vi "NDHX.vi"(1 "NDHX Tube Length (m)":dbl, 2 "Pipe Diameter (m)":dbl, 3 "Air Average Viscosity (Pa-s)":dbl, 4 "Thermal Conductivity of FLiNaK (W/m-K)":dbl, 5 "Air Mass Flow (kg/s)":dbl, 6 "Sec Hot Temp (K)":dbl, 9 "Stack Inner Diameter (m)":dbl, 10 "Cp of FLiNaK (J/kgK)":dbl, 11 "Sec Cold Temp (K)":dbl, 12 "NDHX Tube Diameter (m)":dbl, 13 "NDHX Number of Tubes":dbl, 14 "Air Cold Temperature (K)":dbl, 15 "Thermal Conductivity of Hastealloy N (W/m-K)":dbl, 16 "Air Hot Temperature (K)":dbl, 18 "Cp of Air (J/kgK)":dbl, 19 "Sec Mass Flow (kg/s)":dbl) -> (20 "NDHX Heating Transfer (W)":dbl, 21 "Wall Temperature (K)":dbl, 22 "LMTD (K)":dbl)   [LabVIEW 2019]
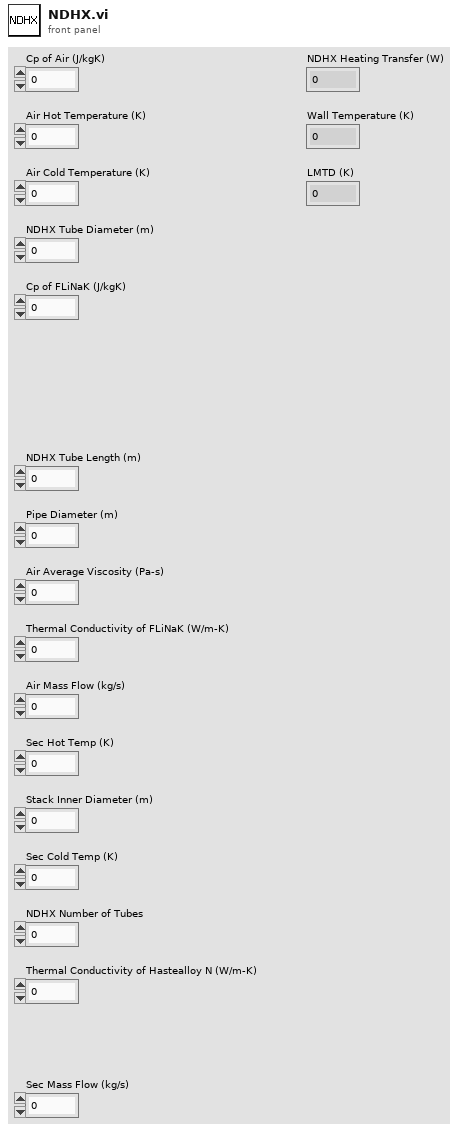
[diagram p1: front panel]
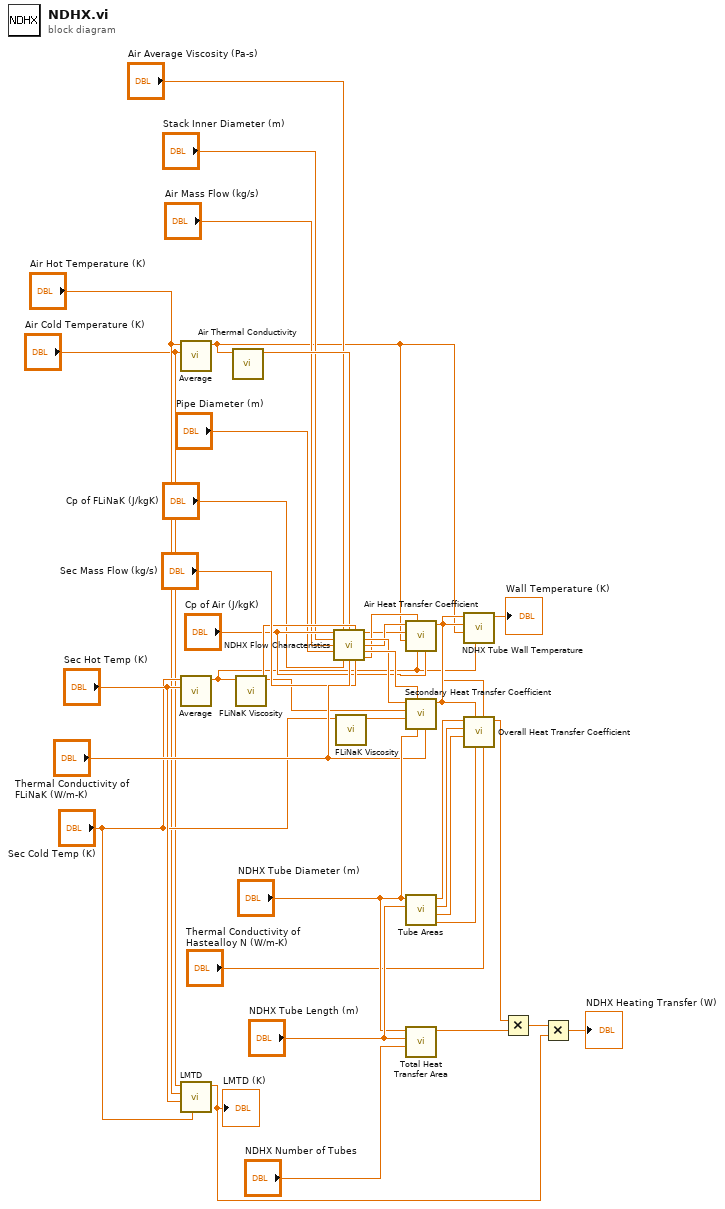
[diagram p0: block diagram]
diagram:
  n1 = call "Average.vi"("Number 2"="Air Cold Temperature (K)", "Number 1"="Air Hot Temperature (K)") -> ("Average"=w1:dbl)  [unwired: 9 in]
  n2 = call "Average.vi"("Number 2"="Sec Hot Temp (K)", "Number 1"="Sec Cold Temp (K)") -> ("Average"=w4:dbl)  [unwired: 9 in]
  n3 = call "LMTD.vi"("Tube Cold Temp (K)"="Sec Cold Temp (K)", "Tube Hot Temp (K)"="Sec Hot Temp (K)", "Shell Hot Temp (K)"="Air Hot Temperature (K)", "Shell Cold Temperature (K)"="Air Cold Temperature (K)") -> ("LMTD (K)"=w37:dbl)  [unwired: 7 in]
  "LMTD (K)" <- w37
  n4 = call "Air Thermal Conductivity.vi"("Temperature (C)"=w1) -> ("Thermal Conductivity (W/m-K)"=w12:dbl)  [unwired: 10 in]
  n5 = call "FLiNaK Viscosity.vi"("Temperature (K)"=w4) -> ("FLiNaK Viscosity (Pa-s)"=w19:dbl)  [unwired: 10 in]
  n6 = call "NDHX Flow Characteristics.vi"("Cp of Air (J/kgK)"="Cp of Air (J/kgK)", "Air Average Viscosity (Pa-s)"="Air Average Viscosity (Pa-s)", "Thermal Conductivity (W/m-K)"=w12, "FLiNaK Viscosity (Pa-s)"=w19, "Stack Inner Diameter"="Stack Inner Diameter (m)", "Air Mass Flow (kg/s)"="Air Mass Flow (kg/s)", "Pipe Diameter (m)"="Pipe Diameter (m)", "Cp of FLiNaK (J/kgK)"="Cp of FLiNaK (J/kgK)", "Thermal Conductivity of FLiNaK (W/m-K)"="Thermal Conductivity of FLiNaK (W/m-K)", "Sec Mass Flow (kg/s)"="Sec Mass Flow (kg/s)") -> ("Air Re"=w13:dbl, "Sec Re"=w17:dbl, "Air Pr"=w16:dbl, "Sec Pr"=w18:dbl, "Air Mass Flux (kg/s-m^2)"=w15:dbl)  [unwired: 1 in]
  n7 = call "FLiNaK Viscosity.vi"("Temperature (K)"="Sec Cold Temp (K)") -> ("FLiNaK Viscosity (Pa-s)"=w20:dbl)  [unwired: 10 in]
  n8 = call "Air Heat Transfer Coefficient.vi"("Cp of Air (J/kgK)"="Cp of Air (J/kgK)", "Wall Temperature (K)"=w4, "Air Mass Flux (kg/s-m^2)"=w15, "Air Temperature (K)"=w1, "Air Re"=w13, "Air Pr"=w16) -> ("Air Heat Xfer Coeff"=w24:dbl)  [unwired: 5 in]
  n9 = call "Secondary Heat Transfer Coefficient.vi"("Thermal Conductivity of FLiNaK (W/m-K)"="Thermal Conductivity of FLiNaK (W/m-K)", "NDHX Tube Diameter (m)"="NDHX Tube Diameter (m)", "Sec Pr"=w18, "FLiNaK Viscosity (Pa-s)"=w20, "FLiNaK Viscosity (Pa-s) 2"=w19, "Sec Re"=w17) -> ("Sec Heat Xfer Coeff"=w28:dbl)  [unwired: 5 in]
  n10 = call "Tube Areas.vi"("NDHX Tube Length (m)"="NDHX Tube Length (m)", "NDHX Tube Diameter (m)"="NDHX Tube Diameter (m)") -> ("Wall Thickness (m)"=w25:dbl, "Am"=w27:dbl, "Ai"=w30:dbl, "Ao"=w29:dbl)  [unwired: 6 in]
  n11 = call "Total Heat Transfer Area.vi"("NDHX Number of Tubes"="NDHX Number of Tubes", "NDHX Tube Length (m)"="NDHX Tube Length (m)", "NDHX Tube Diameter (m)"="NDHX Tube Diameter (m)") -> ("Total Heat Transfer Area (m^2)"=w34:dbl)  [unwired: 8 in]
  n12 = call "NDHX Tube Wall Temperature.vi"("Sec Temperature (K)"=w4, "Air Temperature (K)"=w1, "Air Heat Xfer Coeff"=w24, "Sec Heat Xfer Coeff"=w28) -> ("Wall Temperature (K)"=→"Wall Temperature (K)":dbl)  [unwired: 7 in]
  n13 = call "Overall Heat Transfer Coefficient.vi"("Thermal Conductivity of Hastealloy N (W/m-K)"="Thermal Conductivity of Hastealloy N (W/m-K)", "Air Heat Xfer Coeff"=w24, "Wall Thickness (m)"=w25, "Sec Heat Xfer Coeff"=w28, "Am"=w27, "Ai"=w30, "Ao"=w29) -> ("Overall Heat Xfer Coeff"=w35:dbl)  [unwired: 4 in]
  n14 = Multiply(x=w35, y=w34) -> (x*y=w36:dbl)
  n15 = Multiply(x=w36, y=w37) -> (x*y=→"NDHX Heating Transfer (W)":dbl)
